vi "contains read gain subvi (used in CP).vi"() -> ()   [LabVIEW 2009]
panel:
  out "result string":string
  out "VISA resource name out":refnum<visa-resource-name>
  in  "VISA resource name":refnum<visa-resource-name>="GPIB0::12::INSTR"
  in  "error in (no error)":errorcluster
  out "error out":errorcluster
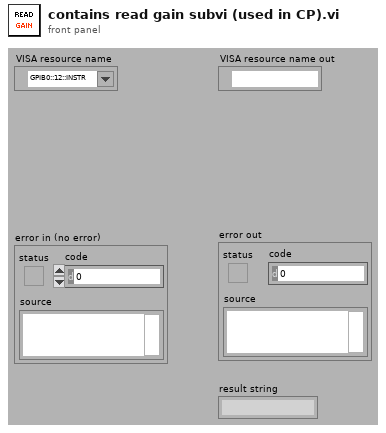
[diagram p1: front panel]
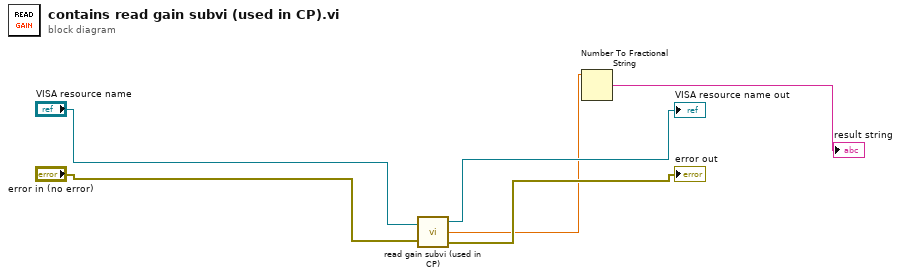
[diagram p0: block diagram]
diagram:
  n1 = call "read gain subvi (used in CP).vi"("VISA resource name"="VISA resource name", "error in (no error)"="error in (no error)") -> ("VISA resource name out"=→"VISA resource name out":refnum<visa-resource-name>, "Gain (%)"=w2:dbl, "error out"=→"error out":errorcluster)
  n2 = Number To Fractional String(number=w2) -> (F-format string=→"result string":string)  [unwired: 3 in]
